vi "Create Certificate and Keys.vi"(8 "error in (no error)":errorcluster, 10 "Set as Active":bool=TRUE, 11 "IoT Session in":refnum<class "IoT Session.lvclass">) -> (0 "error out":errorcluster, 2 "Certificate and Keys":T1, 3 "IoT Session out":refnum<class "IoT Session.lvclass">)   [LabVIEW 2015, in "NI_AWS_IoT.lvlib" / "IoT Session.lvclass"]
uses:
  IoT Session.lvclass
  Certificate and Keys.ctl
  Core/HTTP Request/Request Options.ctl
  Core/HTTP Request/Name Value Pair.ctl
  Core/HTTP Request/Region handling.ctl
  Core/HTTP Request/URL formatting.ctl
  Core/HTTP Request/HTTP Request.lvclass
  JSON Parsing/NI_JSON Parsing.lvlib
  NI_AWS_IoT.lvlib
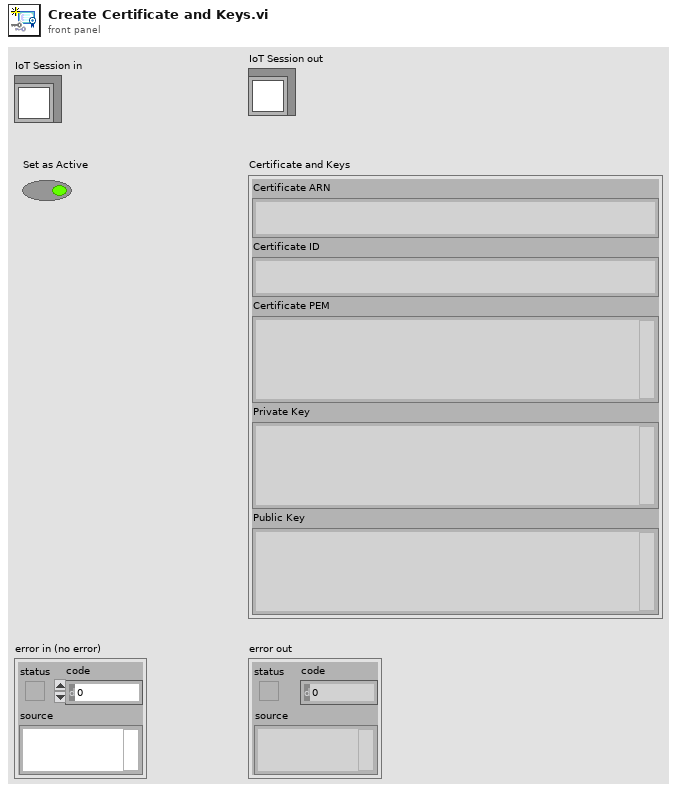
[diagram p1: front panel]
types:
  T1 = typedef "NI_AWS_IoT.lvlib/Certificate and Keys.ctl" = cluster{"Certificate ARN":string, "Certificate ID":string, "Certificate PEM":string, "Private Key":string, "Public Key":string}
  T2 = typedef "NI_AWS_Core.lvlib/HTTP Request.lvclass/Name Value Pair.ctl" = cluster{"name":string, "value":string}
  T3 = typedef "NI_AWS_Core.lvlib/HTTP Request.lvclass/Request Options.ctl" = cluster{"request headers":T2[], "request parameters":T2[], "request body":string, "region handling":T4, "URL formatting":T5}
  T4 = typedef "NI_AWS_Core.lvlib/HTTP Request.lvclass/Region handling.ctl" = enum16{"use region everywhere", "use region (authentication only)", "use region (URL only)", "ignore region everwhere"}
  T5 = typedef "NI_AWS_Core.lvlib/HTTP Request.lvclass/URL formatting.ctl" = enum16{"region-", "region."}
  T6 = typedef "NI_AWS_Core.lvlib/HTTP Request.lvclass/Response.ctl" = cluster{"Headers":string, "Body":string}
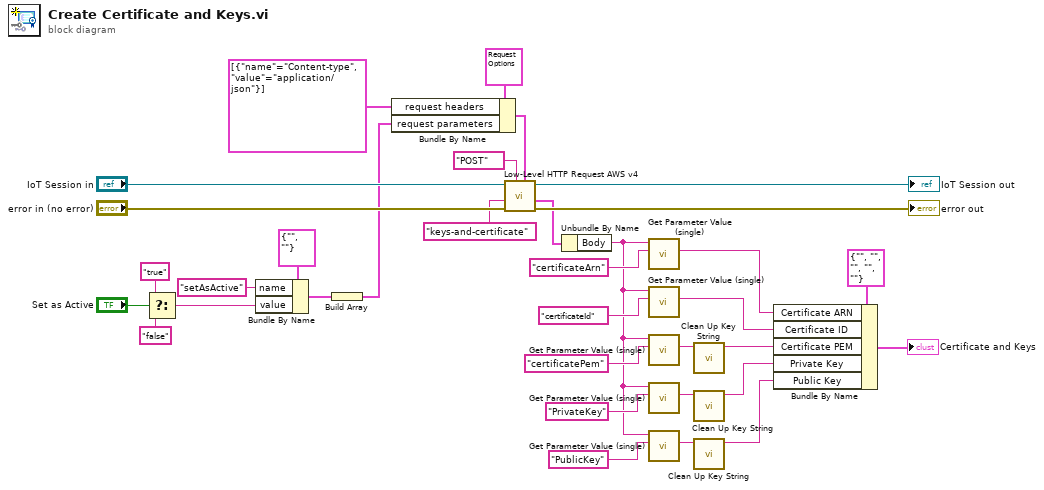
[diagram p0: block diagram]
diagram:
  n1 = Select(t="true", s="Set as Active", f="false") -> (s? t:f=w18:string)
  n2 = Bundle By Name(cluster=T2 {"name"="", "value"=""} ("Name Value Pair"), "name"="setAsActive", "value"=w18) -> (w24:T2)
  n3 = Build Array(w24) -> (w23:T2[])
  n4 = Bundle By Name(cluster=T3 {"request headers"=[], "request parameters"=[], "request body"="", "region handling"=enum."use region everywhere", "URL formatting"=enum."region."} ("Request Options"), "request headers"=T2[] [{"name"="Content-type", "value"="application/json"}], "request parameters"=w23) -> (w27:T3)
  n5 = call "Low-Level HTTP Request AWS v4.vi"("Request Options"=w27, "HTTP-Verb"="POST", "error in (no error)"="error in (no error)", "URL Suffix"="keys-and-certificate", "AWS Core in"="IoT Session in") -> ("error out"=→"error out":errorcluster, "Response"=w17:T6, "AWS Core out"=→"IoT Session out":refnum<class "IoT Session.lvclass">)  [unwired: 3 in, 1 out]
  n6 = Unbundle By Name(w17) -> ("Body"=w8:string)
  n7 = call "Get Parameter Value (single).vi"("Parameter Name"="certificateArn", "JSON"=w8) -> ("Parameter Value"=w13:string)  [unwired: 6 in, 3 out]
  n8 = call "Get Parameter Value (single).vi"("Parameter Name"="certificateId", "JSON"=w8) -> ("Parameter Value"=w7:string)  [unwired: 6 in, 3 out]
  n9 = call "Get Parameter Value (single).vi"("Parameter Name"="certificatePem", "JSON"=w8) -> ("Parameter Value"=w6:string)  [unwired: 6 in, 3 out]
  n10 = call "Get Parameter Value (single).vi"("Parameter Name"="PrivateKey", "JSON"=w8) -> ("Parameter Value"=w5:string)  [unwired: 6 in, 3 out]
  n11 = call "Get Parameter Value (single).vi"("Parameter Name"="PublicKey", "JSON"=w8) -> ("Parameter Value"=w4:string)  [unwired: 6 in, 3 out]
  n12 = call "Clean Up Key String.vi"("Key"=w6) -> ("Cleaned Up Key"=w3:string)  [unwired: 10 in]
  n13 = call "Clean Up Key String.vi"("Key"=w5) -> ("Cleaned Up Key"=w2:string)  [unwired: 10 in]
  n14 = call "Clean Up Key String.vi"("Key"=w4) -> ("Cleaned Up Key"=w1:string)  [unwired: 10 in]
  n15 = Bundle By Name(cluster=T1 {"Certificate ARN"="", "Certificate ID"="", "Certificate PEM"="", "Private Key"="", "Public Key"=""} ("Certificate and Keys"), "Certificate ARN"=w13, "Certificate ID"=w7, "Certificate PEM"=w3, "Private Key"=w2, "Public Key"=w1) -> (→"Certificate and Keys":T1)
